vi "Load LCOS Configuration.vi"(11 "LCOS Configuration Ref":refnum<vi>) -> ()   [LabVIEW 2011]
panel:
  out "Error Out":errorcluster
  in  "Error In":errorcluster
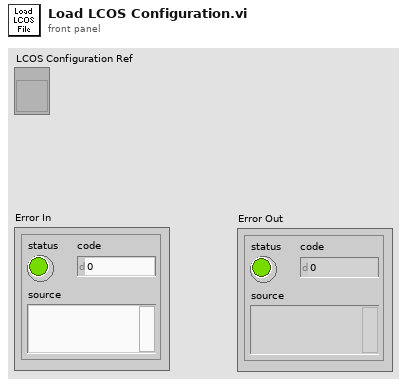
[diagram p1: front panel]
types:
  T1 = typedef "Periodic Spot Pattern Parameters.ctl" = cluster{"X pitch":dbl, "rotation":dbl, "Center H":dbl, "Center V":dbl, "# Spots H":u32, "# Spots V":u32, "Spot size":dbl, "ref_spot _dark":bool, "Exact Phase Formula":bool, "phase_wrap_pos":bool, "Set Focus (mm)":dbl, "phase_max":dbl, "phase_factor":u8, "Steer LW":u32, "Steer vmax":u8, "phase_wrap_neg":bool, "steer_horiz":bool, "steer_pad":i64, "steer_only":bool, "Wavelength":dbl, "Y pitch":dbl, "python":bool, "test_pattern":bool, "grid":bool, "dark_all":bool, "Xm_str":string, "Ym_str":string, "ref_spot":i64, "stretch":bool}
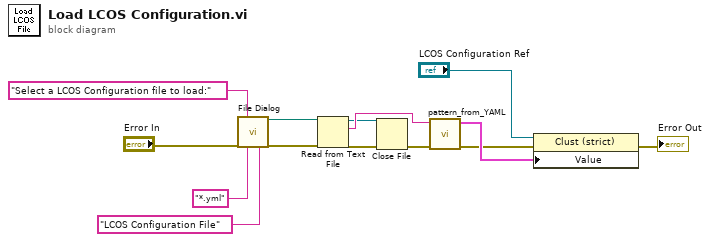
[diagram p0: block diagram]
diagram:
  n1 = call "File Dialog"("prompt"="Select a LCOS Configuration file to load:", "error in"="Error In", "pattern (all files)"="*.yml", "pattern label"="LCOS Configuration File") -> ("selected path"=w9:path, "error out"=w10:errorcluster)  [unwired: 8 in, 2 out]
  n2 = Read from Text File(file (use dialog)=w9, error in=w10) -> (refnum out=w5:refnum<file>, text=w7:string, error out=w6:errorcluster)  [unwired: 2 in, 1 out]
  n3 = Close File(refnum=w5, error in=w6) -> (error out=w4:errorcluster)  [unwired: 1 out]
  n4 = call "pattern_from_YAML.vi"("error in (no error)"=w4, "String"=w7) -> ("error out"=w2:errorcluster, "LCOS Configuration"=w3:T1)  [unwired: 8 in]
  n5 = property class="Clust (strict)"(reference="LCOS Configuration Ref", error in=w2, "Value"=w3) -> (error out=→"Error Out":errorcluster)  [unwired: 1 out]
